vi "C.vi"(10 "Llanta 2":dbl[](array[numeric]), 11 "Llanta 1":dbl[](array[numeric])) -> (3 "Matrix Transpose":T1)   [LabVIEW 2011]
uses:
  <vilib>/Analysis/Matrix/Datatypes/RealMatrix.ctl
  <vilib>/Analysis/7linalg.llb/Real Transpose Matrix.vi
  <vilib>/Analysis/NI_AALPro.lvlib
  <vilib>/Analysis/Matrix/NI_Matrix.lvlib
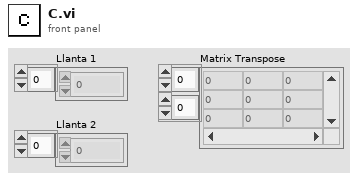
[diagram p1: front panel]
types:
  T1 = typedef "NI_Matrix.lvlib/RealMatrix.ctl" = dbl[][]
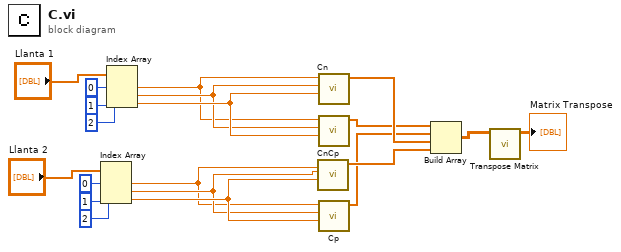
[diagram p0: block diagram]
diagram:
  n1 = Index Array(array="Llanta 2", index #1=0 ("index"), index #2=1 ("index"), index #3=2 ("index")) -> (element #1=w18:dbl, element #2=w19:dbl, element #3=w20:dbl)
  n2 = Index Array(array="Llanta 1", index #1=0 ("index"), index #2=1 ("index"), index #3=2 ("index")) -> (element #1=w8:dbl, element #2=w9:dbl, element #3=w10:dbl)
  n3 = call "Cn.vi"("l"=w20, "beta"=w19, "alpha"=w18) -> ("Array"=w3:dbl[])  [unwired: 8 in]
  n4 = call "Cn.vi"("l"=w10, "beta"=w9, "alpha"=w8) -> ("Array"=w4:dbl[])  [unwired: 8 in]
  n5 = call "Cp.vi"("l"=w10, "beta"=w9, "alpha"=w8) -> ("Array"=w1:dbl[])  [unwired: 8 in]
  n6 = call "Cp.vi"("l"=w20, "beta"=w19, "alpha"=w18) -> ("Array"=w2:dbl[])  [unwired: 8 in]
  n7 = Build Array(w1, w2, w4, w3) -> (w5:T1)
  n8 = call-poly <vilib>:"Transpose Matrix.vi"("Input Matrix"=w5) -> ("Matrix Transpose"=→"Matrix Transpose":T1)  [unwired: 9 in, 1 out]
